vi "Generate_Data.vi"(8 "error in":errorcluster caption="entrée d'erreur") -> (0 "error out":errorcluster caption="sortie d'erreur")   [LabVIEW 2026]
panel:
  out "standard error":string caption="erreur standard"
  out "Command":string
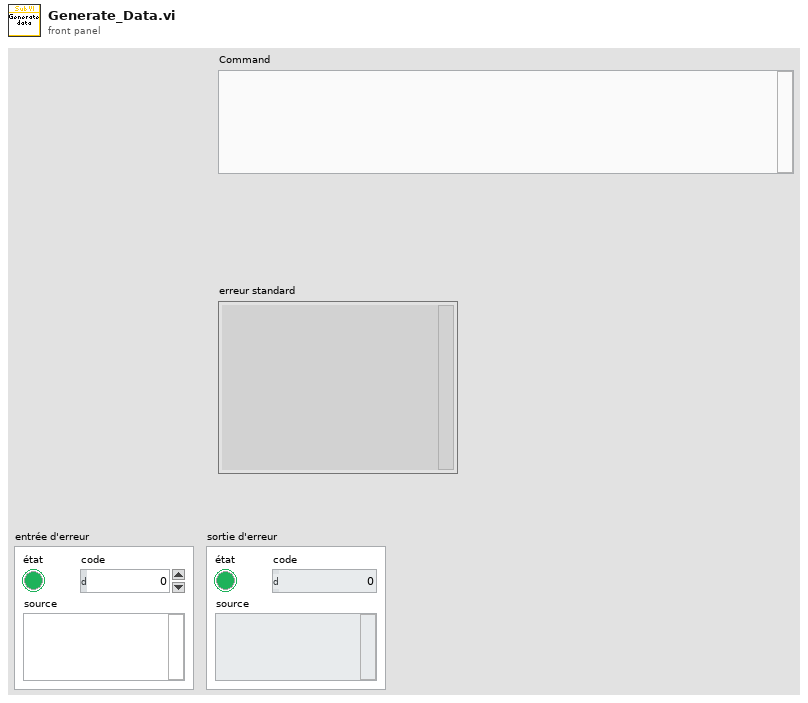
[diagram p1: front panel]
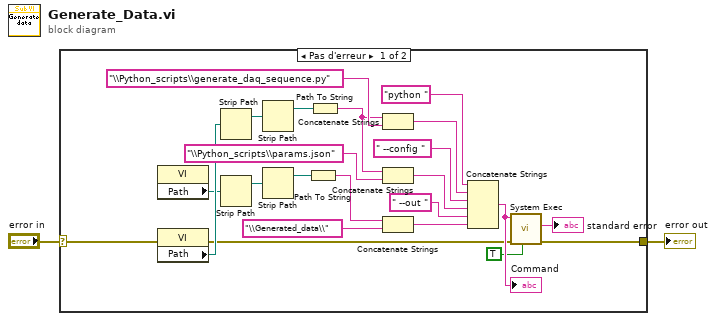
[diagram p0: block diagram]
diagram:
  n1 = case shown="Pas d'erreur" "error in" {
    selector: "error in" -> [w21 w26]
    tunnel: [w6 w26] -> w1
    frame No Error {
      n2 = property class="VI"() -> ("Path"=w17:path)  [unwired: 2 in, 2 out]
      n3 = property class="VI"(error in=w21) -> (error out=w20:errorcluster, "Path"=w22:path)  [unwired: 1 in, 1 out]
      n4 = Strip Path(path=w22) -> (stripped path=w13:path)  [unwired: 1 out]
      n5 = Strip Path(path=w17) -> (stripped path=w5:path)  [unwired: 1 out]
      n6 = Strip Path(path=w13) -> (stripped path=w12:path)  [unwired: 1 out]
      n7 = Strip Path(path=w5) -> (stripped path=w4:path)  [unwired: 1 out]
      n8 = Path To String(path=w4) -> (string=w16:string)
      n9 = Path To String(path=w12) -> (string=w11:string)
      n10 = Concatenate Strings(w11, "\\Python_scripts\\generate_daq_sequence.py" ("Python_file")) -> (w18:string)
      n11 = Concatenate Strings(w11, "\\Python_scripts\\params.json" ("Python_file")) -> (w9:string)
      n12 = Concatenate Strings(w16, "\\Generated_data\\" ("Python_file")) -> (w7:string)
      n13 = Concatenate Strings("python ", w18, " --config " ("chaîne"), w9, " --out " ("chaîne"), w7) -> (w23:string)
      "Command" <- w23
      n14 = call <vilib>:"System Exec.vi"("run minimized? (F)"=TRUE, "error in (no error)"=w20, "command line"=w23) -> ("error out"=w6:errorcluster, "standard error"=→"standard error":string)  [unwired: 5 in, 2 out]
    }
    frame Error {
    }
  }
  "error out" <- w1
